vi "FTW-Supervisor-Core-Construct.vi"(0 "Initialization Sequence":string, 5 "FTW Supervisor Configuration":string, 11 "error in":errorcluster) -> (4 "FTW Supervisor":refnum<class "FTW-Supervisor.lvclass">, 6 "Incoming Request":refnum<event-registration>, 15 "error out":errorcluster)   [LabVIEW 2015, in "FTW-Supervisor.lvclass"]
uses:
  FTW-Supervisor.lvclass
  json/core/FTW-JSON-Core-Structure.ctl
  database/core/FTW-SQLite-Core-AccessMode.ctl
  FTW-Supervisor.lvclass/FTW-Supervisor.ctl
  error/FTW-ERR-ThrowError.vi
  reflection/FTW-Reflection-Type.vi
  error/FTW-ERR-NoErrorConstant.vi
  error/FTW-ERR-CallChain.vi
  string/FTW-STR-ReplaceWhitespace.vi
  reflection/FTW-Reflection-Array.vi
  string/FTW-STR-Array-Delimit.vi
  error/FTW-ERR-Clear.vi
  regex/FTW-Regex-ReplaceAll.vi
  lib/FTW-KernelFilepath.vi
  json/core/FTW-JSON-Core-EncodingFlags.vi
  codegen/xnode/json/fetch/FTW-JSON-Core-GetFlattenedValue.vi
  codegen/xnode/FTW-JSON-Fetch.xnode
  instance/FTW-Actor-Instance.lvclass
panel:
  # "Inputs"
  # "Outputs"
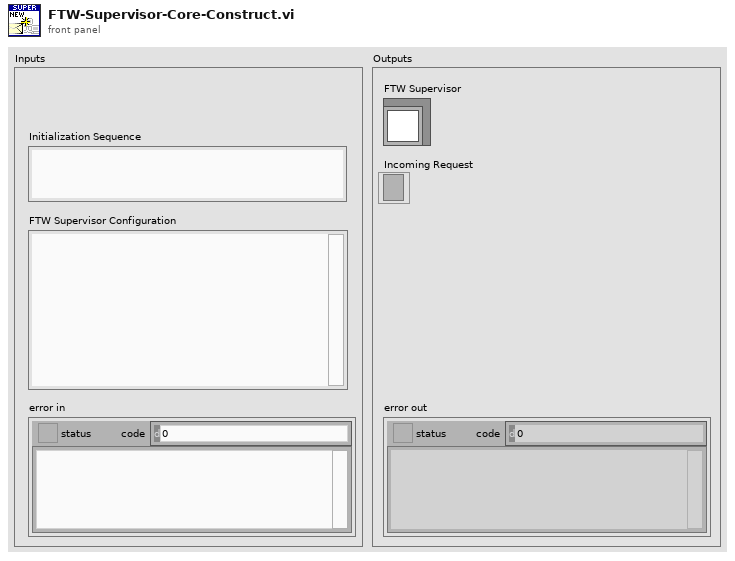
[diagram p1: front panel]
types:
  T1 = typedef "FTW-SQLite-Core-AccessMode.ctl" = enum16{"Read", "Read/Write", "Read/Write/Create"}
  T2 = cluster{"AppName":string, "AppVersionMajor":u32, "AppVersionMinor":u32, "AppVersionPatch":u32, "DashboardInboxAddress":string, "DashboardPublisherAddress":string, "DashboardPageAddress":string, "LogRetentionPolicy":cluster{"PersistToDisk":bool, "LogFilepath":path}}
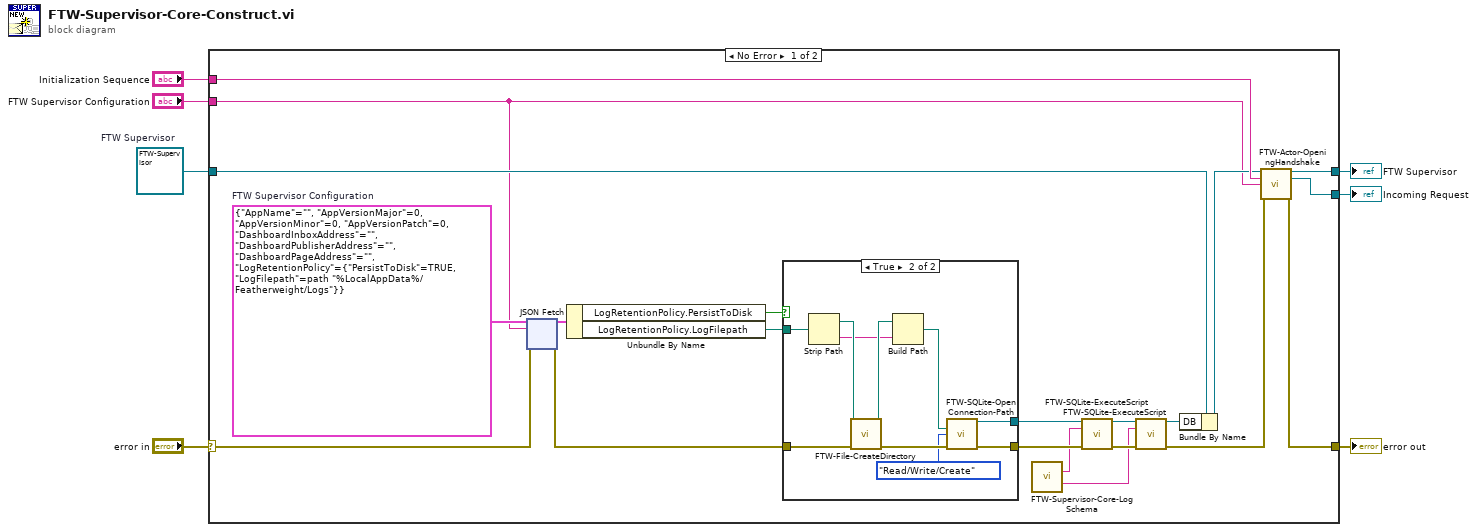
[diagram p0: block diagram]
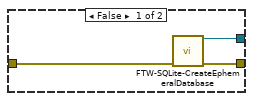
[diagram p2: hidden frame]
diagram:
  w7 = refnum<class "FTW-Supervisor.lvclass"> refnum  # FTW Supervisor
  n1 = case shown="No Error" "error in" {
    selector: "error in" -> [w9 w104]
    tunnel: [w26 w104] -> w5
    tunnel: [w28 w103] -> w1
    tunnel: w7 -> [w24 w103]
    tunnel: "FTW Supervisor Configuration" -> [w8 _]
    tunnel: [w27 _] -> w3
    tunnel: "Initialization Sequence" -> [w25 _]
    frame No Error {
      w12 = T2 {"AppName"="", "AppVersionMajor"=0, "AppVersionMinor"=0, "AppVersionPatch"=0, "DashboardInboxAddress"="", "DashboardPublisherAddress"="", "DashboardPageAddress"="", "LogRetentionPolicy"={"PersistToDisk"=TRUE, "LogFilepath"=path "%LocalAppData%/Featherweight/Logs"}}  # FTW Supervisor Configuration
      n2 = xnode "JSON Fetch"("Type and Defaults"=w12, "JSON String"=w8, "error in"=w9) -> ("Values"=w11:T2, "error out"=w10:errorcluster)  [unwired: 1 in]
      n3 = Unbundle By Name(w11) -> ("LogRetentionPolicy.PersistToDisk"=w22:bool, "LogRetentionPolicy.LogFilepath"=w23:path)
      n4 = case shown="True" w22 {
        tunnel: w10 -> [w90 w102]
        tunnel: [w92 w101] -> w20
        tunnel: [w91 w99] -> w19
        tunnel: w23 -> [_ w97]
        frame False {
          n5 = call "FTW-SQLite-CreateEphemeralDatabase.vi"("error in"=w90) -> ("SQLite Connection"=w92:refnum<data-value>, "error out"=w91:errorcluster)  [unwired: 13 in]
        }
        frame True {
          n6 = Strip Path(path=w97) -> (stripped path=w96:path, name=w93:string)
          n7 = call "FTW-File-CreateDirectory.vi"("Directory to Create"=w96, "error in"=w102) -> ("Created Directory"=w95:path, "error out"=w100:errorcluster)  [unwired: 12 in]
          n8 = Build Path(base path=w95, name or relative path=w93) -> (appended path=w94:path)
          n9 = call "FTW-SQLite-OpenConnection-Path.vi"("Database Filepath"=w94, "Access Mode"=FTW-SQLite-Core-AccessMode."Read/Write/Create", "error in"=w100) -> ("SQLite Connection"=w101:refnum<data-value>, "error out"=w99:errorcluster)  [unwired: 11 in]
        }
      }
      n10 = call "FTW-Supervisor-Core-LogSchema.vi"() -> ("Schema"=w18:string, "Indexes"=w13:string)  [unwired: 14 in]
      n11 = call "FTW-SQLite-ExecuteScript.vi"("SQLite Connection"=w20, "SQL Script"=w18, "error in"=w19) -> ("SQLite Connection out"=w14:refnum<data-value>, "error out"=w16:errorcluster)  [unwired: 10 in, 1 out]
      n12 = call "FTW-SQLite-ExecuteScript.vi"("SQLite Connection"=w14, "SQL Script"=w13, "error in"=w16) -> ("SQLite Connection out"=w17:refnum<data-value>, "error out"=w15:errorcluster)  [unwired: 10 in, 1 out]
      n13 = Bundle By Name(cluster=w24, "DB"=w17) -> (w21:refnum<class "FTW-Supervisor.lvclass">)
      n14 = call "FTW-Actor-OpeningHandshake.vi"("FTW Actor Instance Type"=w21, "Initialization Job Sequence"=w25, "Actor Instance Configuration"=w8, "error in"=w15) -> ("FTW Actor Instance"=w28:refnum<class "FTW-Supervisor.lvclass">, "Incoming Request"=w27:refnum<event-registration>, "error out"=w26:errorcluster)  [unwired: 9 in]
    }
    frame Error {
    }
  }
  "error out" <- w5
  "FTW Supervisor" <- w1
  "Incoming Request" <- w3
